vi "Pressure Setpoint SI.vi"(7 "Set? (F:Read)":bool, 8 "Error In":errorcluster, 9 "Pressure Setpoint (0 hPa)":dbl[unit], 11 "VISA resource name":refnum<visa-resource-name>) -> (0 "Error Out":errorcluster, 1 "Pressure Setpoint out":dbl[unit], 3 "dup VISA resource name":refnum<visa-resource-name>)   [LabVIEW 2011, in "MGC647C.lvlib"]
doc: "Read/Set pressure setpoint in SI unit."
uses:
  <instrlib>/MGC647C/MGC647C.lvlib
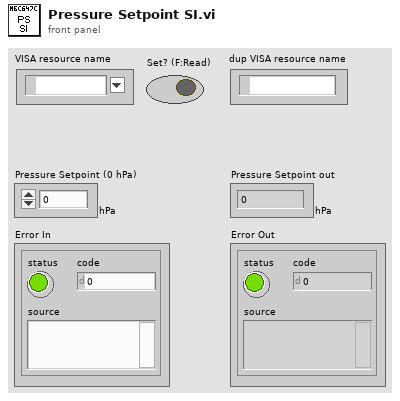
[diagram p1: front panel]
types:
  T1 = enum16{"1.0000 mTorr", "10.000 mTorr", "100.00 mTorr", "1000.0 mTorr", "1.0000 Torr", "10.000 Torr", "100.00 Torr", "1000.0 Torr", "1.0000 kTorr", "10.000 kTorr", "100.00 kTorr", "1.0000 µBar", "10.000 µBar", "100.00 µBar", "1000.0 µBar", "1.0000 mBar", "10.000 mBar", "100.00 mBar", "1000.0 mBar", "1.0000 Bar", "10.000 Bar", "100.00 Bar", "1.0000 Pa", "10.000 Pa", "100.00 Pa", "1.0000 kPa", "10.000 kPa", "100.00 kPa", "1000.0 kPa"}
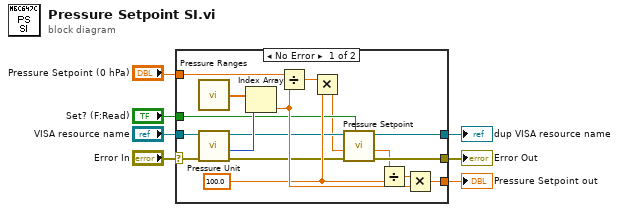
[diagram p0: block diagram]
diagram:
  n1 = case shown="No Error" "Error In" {
    selector: "Error In" -> [w17 w26]
    tunnel: "VISA resource name" -> [w18 w25]
    tunnel: [w12 w25] -> w6
    tunnel: [w11 w26] -> w5
    tunnel: "Set? (F:Read)" -> [w10 _]
    tunnel: "Pressure Setpoint (0 hPa)" -> [w22 w27]
    tunnel: [w23 w27] -> w1
    frame No Error {
      w19 = 100.0 ("y")
      n2 = call <instrlib>:"Pressure Ranges.vi"() -> ("Pressure Ranges"=w15:dbl[unit][])
      n3 = call <instrlib>:"Pressure Unit.vi"("Error In"=w17, "VISA resource name"=w18) -> ("Error Out"=w13:errorcluster, "Unit out"=w16:T1, "dup VISA resource name"=w14:refnum<visa-resource-name>)  [unwired: 7 in]
      n4 = Index Array(array=w15, index=w16) -> (element=w21:dbl[unit])
      n5 = Divide(x=w22, y=w21) -> (x/y=w20:dbl)
      n6 = Multiply(x=w20, y=w19) -> (x*y=w9:dbl)
      n7 = call <instrlib>:"Pressure Setpoint.vi"("Set? (F:Read)"=w10, "Error In"=w13, "Pressure Setpoint (0%)"=w9, "VISA resource name"=w14) -> ("Error Out"=w11:errorcluster, "Pressure Setpoint out"=w8:dbl, "dup VISA resource name"=w12:refnum<visa-resource-name>)  [unwired: 5 in]
      n8 = Divide(x=w8, y=w19) -> (x/y=w24:dbl)
      n9 = Multiply(x=w24, y=w21) -> (x*y=w23:dbl[unit])
    }
    frame Error {
    }
  }
  "dup VISA resource name" <- w6
  "Error Out" <- w5
  "Pressure Setpoint out" <- w1
